vi "PDC_GetMaxPartition.vi"(8 "error in (no error)":errorcluster, 10 "ChildNo":u32, 11 "DeviceNo":u32) -> (0 "error out":errorcluster, 1 "Block":u32, 2 "Count":u32, 3 "ReturnValue":u32, 4 "ErrorCode":u32)   [LabVIEW 2015]
doc: "This VI retrieves the maximum number of divided partitions and the maximum number of blocks in the specified child device."
uses:
  PDCLIB.dll
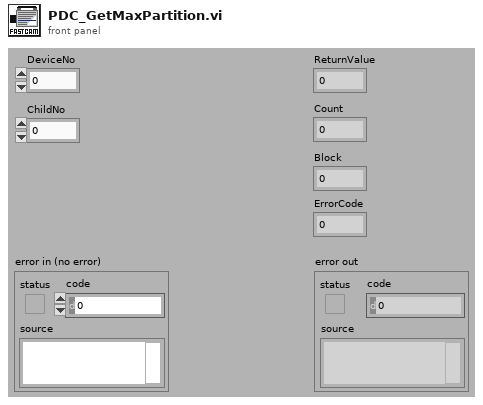
[diagram p1: front panel]
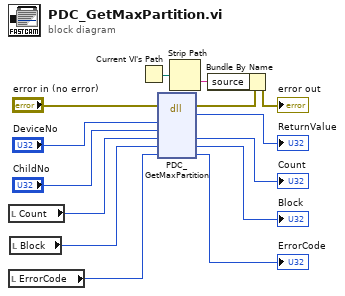
[diagram p0: block diagram]
diagram:
  n1 = local read "Count"() -> (w7:u32)
  n2 = local read "ErrorCode"() -> (w11:u32)
  n3 = local read "Block"() -> (w6:u32)
  n4 = Current VI's Path() -> (path=w3:path)
  n5 = dll-call lib="PDCLIB.dll" fn="PDC_GetMaxPartition"(error in="error in (no error)", "nDeviceNo"="DeviceNo", "nChildNo"="ChildNo", "pCount"=w7, "pBlock"=w6, "pErrorCode"=w11) -> (error out=w2:errorcluster, "return type"=→"ReturnValue":u32, "pCount"=→"Count":u32, "pBlock"=→"Block":u32, "pErrorCode"=→"ErrorCode":u32)  [unwired: 4 in, 1 out]
  n6 = Strip Path(path=w3) -> (name=w4:string)  [unwired: 1 out]
  n7 = Bundle By Name(cluster=w2, "source"=w4) -> (→"error out":errorcluster)
